vi "Report Error.vi"(8 "error in (no error)":errorcluster, 9 "Message":string, 11 "Task in":refnum<class "Task.lvclass">) -> (0 "error out":errorcluster, 3 "Task out":refnum<class "Task.lvclass">)   [LabVIEW 2020, in "Volatus.lvlib" / "Task.lvclass"]
uses:
  Task.lvclass
  Task.lvclass/Task.ctl
  Event API/EventAPI.lvclass/EventAPI.ctl
  EventHandler Messages/Handle Event Msg/Handle Event Msg.lvclass/Handle Event Msg.ctl
  <vilib>/ActorFramework/Message Enqueuer/Message Enqueuer.lvclass/Message Enqueuer.ctl
  Event API/Report Event.vi
  EventHandler Messages/Handle Event Msg/Send Handle Event.vi
  <vilib>/ActorFramework/Message Enqueuer/Enqueue.vi
  EventHandler Messages/Handle Event Msg/Handle Event Msg.lvclass
  C:/Program Files (x86)/National Instruments/LabVIEW 2020/vi.lib/ActorFramework/Message/Message.lvclass
  <vilib>/ActorFramework/Message Priority Queue/Priority Enqueue.vi
  VolatusAPI/VolatusAPI.lvclass
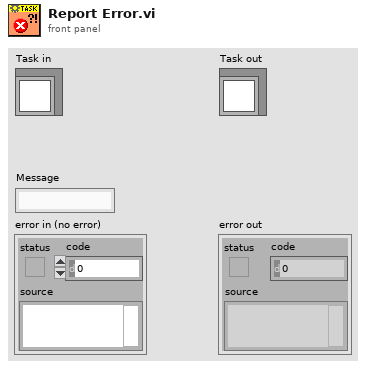
[diagram p1: front panel]
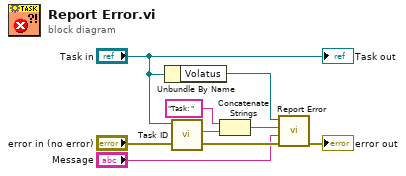
[diagram p0: block diagram]
diagram:
  n1 = Unbundle By Name("Task in") -> ("Volatus"=w8:refnum<class "VolatusAPI.lvclass">)
  n2 = call-dynamic "Task ID.vi"("Task in"="Task in") -> ("Task ID"=w4:string)  [unwired: 8 in, 2 out]
  n3 = Concatenate Strings("Task: ", w4) -> (w1:string)
  n4 = call "Report Error.vi"("error in (no error)"="error in (no error)", "Message"="Message", "Context"=w1, "VolatusAPI in"=w8) -> ("error out"=→"error out":errorcluster)  [unwired: 6 in, 1 out]
  "Task out" <- "Task in"
